vi "Create Graphs.vi"(0 "Speed Graph Time":dbl, 1 "Speed":dbl, 2 "Time Delay":dbl, 3 "Error Graph Time":dbl, 4 "Error":dbl) -> (5 "Speed":cluster{dbl, dbl, dbl[]}, 6 "Error":cluster{dbl, dbl, dbl[]})   [LabVIEW 2011]
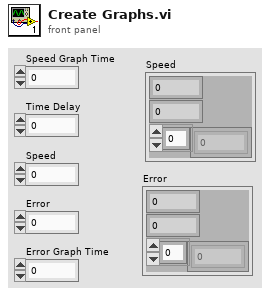
[diagram p1: front panel]
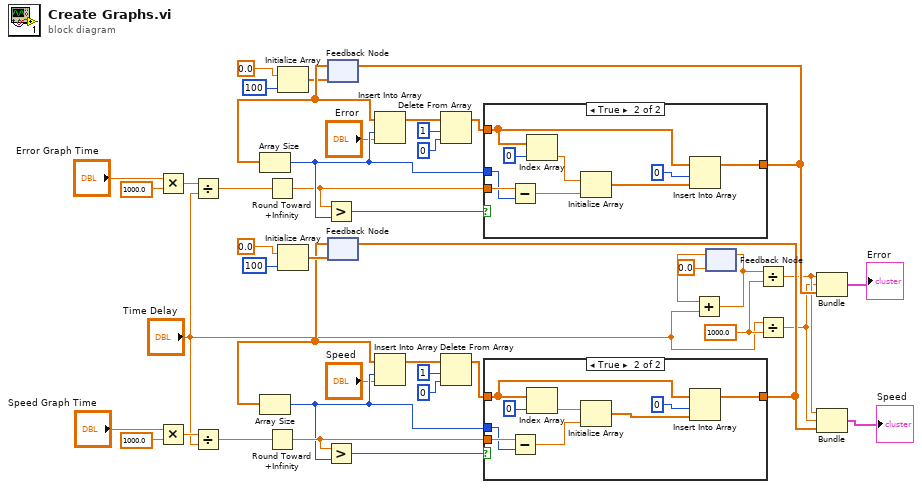
[diagram p0: block diagram]
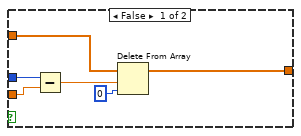
[diagram p2: hidden frame]
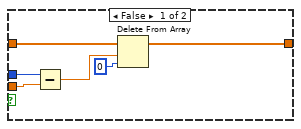
[diagram p3: hidden frame]
diagram:
  w26 = 1000.0 ("y")
  n1 = Multiply(x="Error Graph Time", y=1000.0) -> (x*y=w7:dbl)
  n2 = Multiply(x="Speed Graph Time", y=1000.0) -> (x*y=w29:dbl)
  n3 = Divide(x=w7, y="Time Delay") -> (x/y=w3:dbl)
  n4 = Divide(x=w29, y="Time Delay") -> (x/y=w28:dbl)
  n5 = Round Toward +Infinity(x=w3) -> (ceil(x): smallest int >= x=w20:dbl)
  n6 = Round Toward +Infinity(x=w28) -> (ceil(x): smallest int >= x=w34:dbl)
  n7 = Initialize Array(0.0 ("element"), 100 ("dimension size")) -> (w11:dbl[])
  n8 = Initialize Array(0.0 ("element"), 100 ("dimension size")) -> (w43:dbl[])
  n9 = feedback #1(w11) -> (w14:dbl[])
  n10 = Array Size(array=w14) -> (size(s)=w21:i32)
  n11 = Greater?(x=w20, y=w21) -> (0:w18:bool)
  n12 = feedback #2(w43) -> (w40:dbl[])
  n13 = Array Size(array=w40) -> (size(s)=w33:i32)
  n14 = Greater?(x=w34, y=w33) -> (0:w36:bool)
  n15 = Insert Into Array(array=w14, index=w21, new element="Error") -> (w15:dbl[])
  n16 = Insert Into Array(array=w40, index=w33, new element="Speed") -> (w39:dbl[])
  n17 = Delete From Array(array=w15, length=1, index=0) -> (array with subset deleted=w19:dbl[])  [unwired: 1 out]
  n18 = Delete From Array(array=w39, length=1, index=0) -> (array with subset deleted=w35:dbl[])  [unwired: 1 out]
  n19 = case shown="True" w18 {
    tunnel: w19 -> [w45 w57]
    tunnel: w20 -> [w47 w55]
    tunnel: w21 -> [w48 w54]
    tunnel: [w44 w50] -> w22
    frame False {
      n20 = Subtract(x=w48, y=w47) -> (x-y=w46:dbl)
      n21 = Delete From Array(array=w45, length=w46, index=0) -> (array with subset deleted=w44:dbl[])  [unwired: 1 out]
    }
    frame True {
      n22 = Subtract(x=w55, y=w54) -> (x-y=w53:dbl)
      n23 = Index Array(array=w57, index=0) -> (element=w58:dbl)
      n24 = Initialize Array(w58, w53) -> (w52:dbl[])
      n25 = Insert Into Array(array=w57, index=0, new element=w52) -> (w50:dbl[])
    }
  }
  n26 = feedback-in #1(w22) -> ()
  n27 = case shown="True" w36 {
    tunnel: w35 -> [w60 w72]
    tunnel: w34 -> [w62 w70]
    tunnel: w33 -> [w63 w69]
    tunnel: [w59 w65] -> w32
    frame False {
      n28 = Subtract(x=w63, y=w62) -> (x-y=w61:dbl)
      n29 = Delete From Array(array=w60, length=w61, index=0) -> (array with subset deleted=w59:dbl[])  [unwired: 1 out]
    }
    frame True {
      n30 = Subtract(x=w70, y=w69) -> (x-y=w68:dbl)
      n31 = Index Array(array=w72, index=0) -> (element=w73:dbl)
      n32 = Initialize Array(w73, w68) -> (w67:dbl[])
      n33 = Insert Into Array(array=w72, index=0, new element=w67) -> (w65:dbl[])
    }
  }
  n34 = feedback-in #2(w32) -> ()
  n35 = feedback #3(0.0) -> (w24:dbl)
  n36 = Add(x=w24, y="Time Delay") -> (x+y=w25:dbl)
  n37 = feedback-in #3(w25) -> ()
  n38 = Divide(x=w25, y=w26) -> (x/y=w9:dbl)
  n39 = Divide(x="Time Delay", y=w26) -> (x/y=w8:dbl)
  n40 = Bundle(w9, w8, w22) -> (→"Error":cluster{dbl, dbl, dbl[]})  [unwired: 1 in]
  n41 = Bundle(w9, w8, w32) -> (→"Speed":cluster{dbl, dbl, dbl[]})  [unwired: 1 in]
